vi "3201告警信息改变发送 (子VI).vi"(8 "错误输入":errorcluster caption="错误输出") -> (0 "错误输出":errorcluster)   [LabVIEW 2016, in "数据传输系统-06.lvlib"]
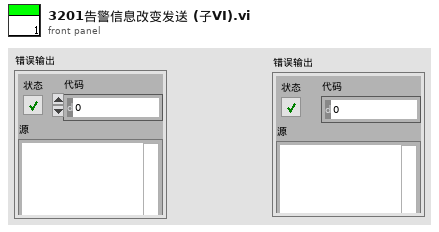
[diagram p1: front panel]
types:
  T1 = cluster{"温度告警":u16, "湿度告警":u16, "烟感告警":u16, "水浸告警":u16, "门禁告警":u16}
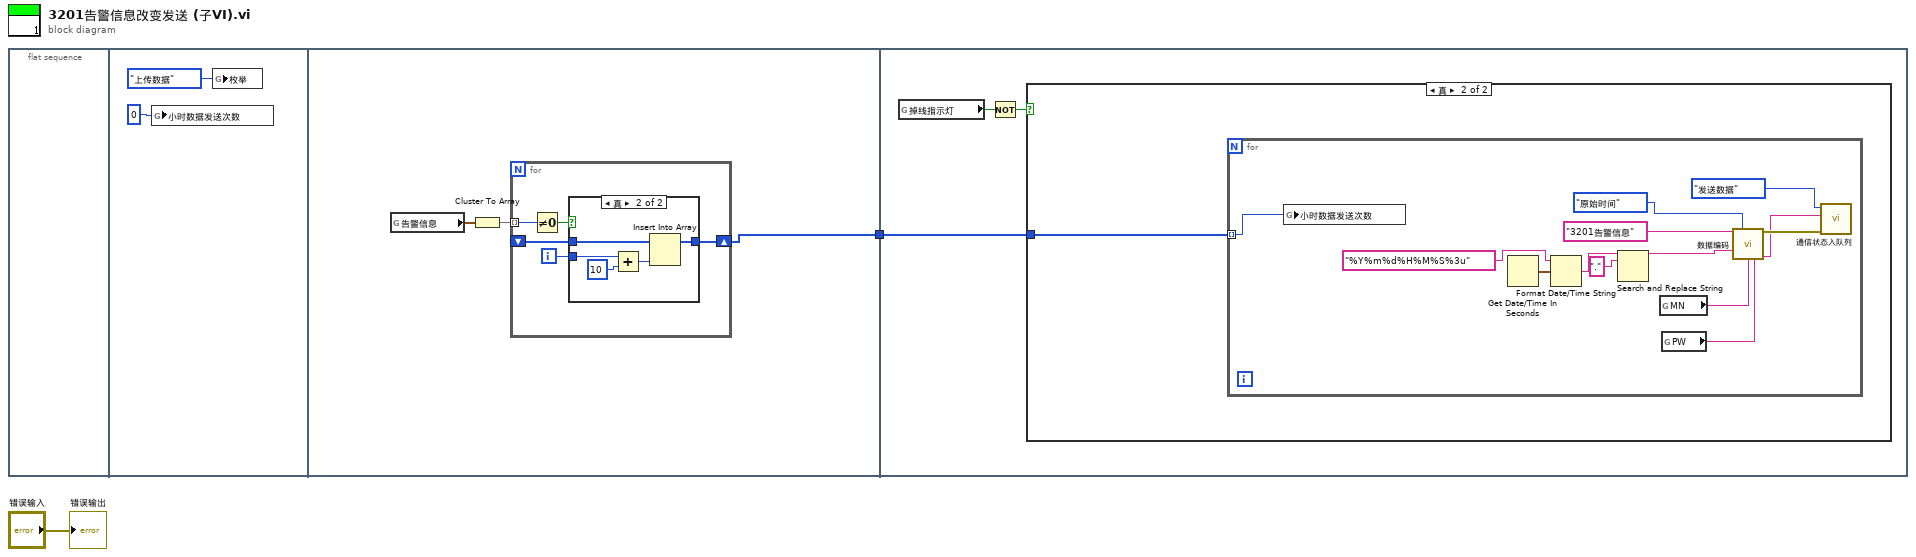
[diagram p0: block diagram]
diagram:
  n1 = flat-sequence {
    tunnel: [w5] -> w1
    tunnel: w1 -> [w19]
    frame #0 {
    }
    frame #1 {
      n2 = global write "全局 小时数据发送次数.vi" "小时数据发送次数"(0 ("小时数据发送次数")) -> ()
      n3 = global write "全局1.vi" "枚举"(enum16{"返回请求应答", "上传数据", "返回执行结果"}."上传数据" ("枚举")) -> ()
    }
    frame #2 {
      n4 = global read "全局1.vi" "告警信息"() -> (w7:T1)
      n5 = Cluster To Array(cluster=w7) -> (array=w6:u16[])
      n6 = for {
        tunnel: w6 -> [w12] mode=indexing
        shift-right: [w8] -> w5
        shift-left: _ -> [w9]
        i -> [w11]
        n7 = Not Equal To 0?(x=w12) -> (x != 0?=w10:bool)
        n8 = case shown="真" w10 {
          tunnel: w11 -> [_ w16]
          tunnel: w9 -> [w13 w18]
          tunnel: [w13 w17] -> w8
          frame False {
          }
          frame True {
            n9 = Add(x=w16, y=10) -> (x+y=w14:i32)
            n10 = Insert Into Array(array=w18, new element=w14) -> (w17:i32[])  [unwired: 1 in]
          }
        }
      }
    }
    frame #3 {
      n11 = global read "全局 数据发送重叠.vi" "掉线指示灯"() -> (w21:bool)
      n12 = Not(x=w21) -> (.not. x?=w20:bool)
      n13 = case shown="真" w20 {
        tunnel: w19 -> [_ w22]
        frame False {
        }
        frame True {
          n14 = for {
            tunnel: w22 -> [w23] mode=indexing
            n15 = global write "全局 小时数据发送次数.vi" "小时数据发送次数"(w23) -> ()
            n16 = Get Date/Time In Seconds() -> (seconds since 1Jan1904=w33:timestamp)
            n17 = Format Date/Time String(time format string (%c)="%Y%m%d%H%M%S%3u" ("时间格式字符串(%c)"), seconds (now)=w33) -> (date/time string=w32:string)  [unwired: 1 in]
            n18 = Search and Replace String(input string=w32, search string="." ("搜索字符串")) -> (result string=w30:string)  [unwired: 6 in, 3 out]
            n19 = global read "断电保存全局.vi" "MN"() -> (w29:string)
            n20 = global read "断电保存全局.vi" "PW"() -> (w28:string)
            n21 = call "数据编码.vi"("table输入"="3201告警信息" ("新元素/子数组"), "仪器参数上传时间"=enum16{"精确到小时", "原始时间"}."原始时间", "QN"=w30, "MN"=w29, "PW"=w28) -> ("错误常量"=w27:errorcluster, "通讯包字符串"=w24:string)  [unwired: 9 in]
            n22 = call "通信状态入队列.vi"("错误输入（无错误）"=w27, "发送报文"=w24, "枚举"=enum16{"打开连接", "发送数据", "读取数据", "数据处理", "关闭连接"}."发送数据") -> ()  [unwired: 8 in, 1 out]
          }
        }
      }
    }
  }
  "错误输出" <- "错误输入"
